vi "Motor Set Output (Shooter Speed).vi"(6 "Isochronous":bool, 8 "error in (no error)":errorcluster, 9 "Sync Group":u8, 10 "Output":dbl, 11 "MotorControlDevRef":cluster{string, i32}) -> (0 "error out":errorcluster, 2 "Motor Output":dbl, 3 "MotorControlDevRef":cluster{string, i32})   [LabVIEW 2013]
uses:
  Shooter Speed Global.vi
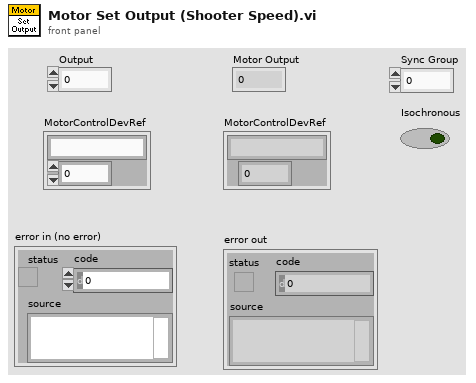
[diagram p1: front panel]
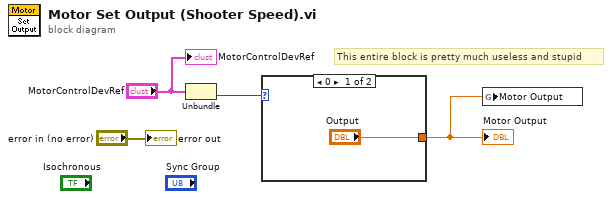
[diagram p0: block diagram]
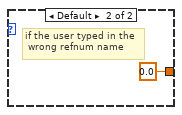
[diagram p2: hidden frame]
diagram:
  # "This entire block is pretty much useless and stupid"
  n1 = Unbundle("MotorControlDevRef") -> (w2:i32)  [unwired: 1 out]
  n2 = case shown="0" w2 {
    tunnel: ["Output" 0.0 ("Output")] -> w1
    frame 0 {
    }
    frame Default {
      # "if the user typed in the\n wrong refnum name"
    }
  }
  "Motor Output" <- w1
  n3 = global write "Shooter Speed Global.vi" "Motor Output"(w1) -> ()
  "error out" <- "error in (no error)"
  "MotorControlDevRef" <- "MotorControlDevRef"
